vi "风扇标志位.vi"(7 "Value":variant, 8 "索引":i32, 9 "类别":string, 11 "vi refnum":refnum<vi>) -> ()   [LabVIEW 2015]
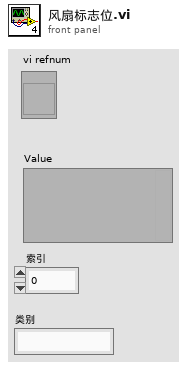
[diagram p1: front panel]
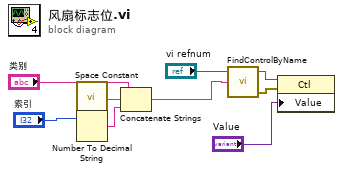
[diagram p0: block diagram]
diagram:
  n1 = call <vilib>:"Space Constant.vi"() -> ("String"=w9:string)
  n2 = Number To Decimal String(number="索引") -> (decimal integer string=w8:string)  [unwired: 1 in]
  n3 = Concatenate Strings("类别", w9, w8) -> (w3:string)
  n4 = call "FindControlByName.vi"("control name"=w3, "vi refnum"="vi refnum") -> ("error out"=w1:errorcluster, "control refnum"=w2:refnum<vi>)  [unwired: 2 in]
  n5 = property class="Ctl"(reference=w2, error in=w1, "Value"="Value") -> ()  [unwired: 2 out]
